vi "Boiler System Open.vi"(8 "error constant":errorcluster) -> (0 "error out":errorcluster, 1 "Configuration Data":T1, 2 "Notifiers":T5, 3 "Message Queues out":T6, 5 "User Event - Stop":refnum<user-event>, 7 "Stop Event Registration Refnum":refnum<event-registration>)   [LabVIEW 2017]
uses:
  Message Queue/All Message Queues.ctl
  Message Queue/Message Cluster.ctl
  Notifieres/Notifiers.ctl
  Configuration/Configuration Data.ctl
  controls/MHL Configuration.ctl
  Controller/Controller Configuration.ctl
  Boiler/Boiler Configuration.ctl
  User Event - Stop/User Event - Stop.lvlib
  Message Queue/Message Queue.lvlib
  Controller/Controller.lvlib
  Boiler/Boiler.lvlib
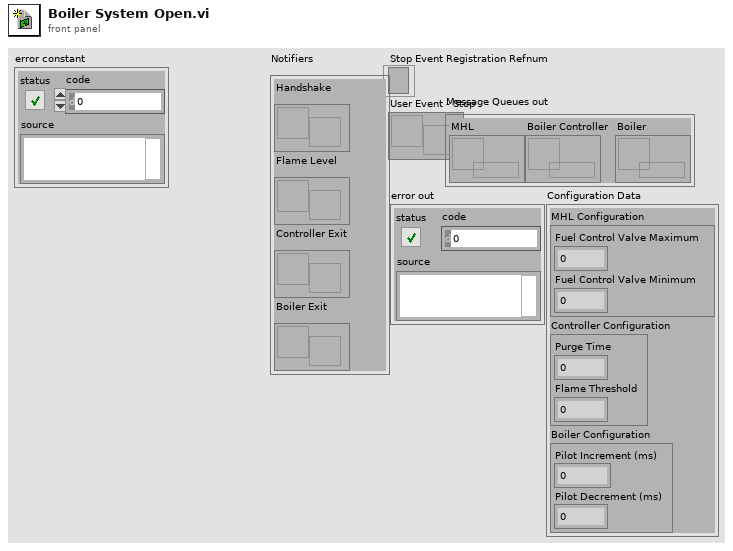
[diagram p1: front panel]
types:
  T1 = typedef "Configuration Data.ctl" = cluster{"MHL Configuration":T2, "Controller Configuration":T3, "Boiler Configuration":T4}
  T2 = typedef "MHL Configuration.ctl" = cluster{"Fuel Control Valve Maximum":dbl, "Fuel Control Valve Minimum":dbl}
  T3 = typedef "Controller.lvlib/Controller Configuration.ctl" = cluster{"Purge Time":u32, "Flame Threshold":u32}
  T4 = typedef "Boiler.lvlib/Boiler Configuration.ctl" = cluster{"Pilot Increment (ms)":u32, "Pilot Decrement (ms)":u32}
  T5 = typedef "Notifiers.ctl" = cluster{"Handshake":refnum<notifier>, "Flame Level":refnum<notifier>, "Controller Exit":refnum<notifier>, "Boiler Exit":refnum<notifier>}
  T6 = typedef "Message Queue.lvlib/All Message Queues.ctl" = cluster{"MHL":refnum<queue>, "Boiler Controller":refnum<queue>, "Boiler":refnum<queue>}
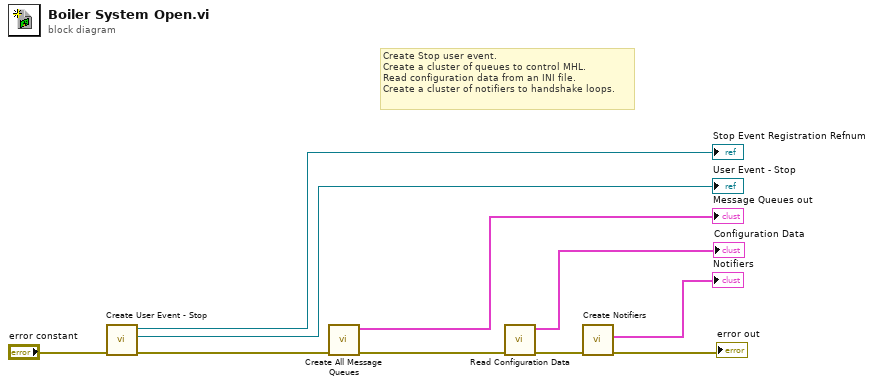
[diagram p0: block diagram]
diagram:
  # "Create Stop user event.\nCreate a cluster of queues to control MHL.\nRead configuration data from an INI file.\nCreate a cluster of notifiers to handshake loops."
  n1 = call "Create User Event - Stop.vi"("error in (no error)"="error constant") -> ("error out"=w7:errorcluster, "User Event - Stop"=→"User Event - Stop":refnum<user-event>, "Stop Event Registration Refnum"=→"Stop Event Registration Refnum":refnum<event-registration>)  [unwired: 8 in]
  n2 = call "Create All Message Queues.vi"("error in (no error)"=w7) -> ("error out"=w3:errorcluster, "Message Queues out"=→"Message Queues out":T6)  [unwired: 9 in]
  n3 = call "Read Configuration Data.vi"("error in (no error)"=w3) -> ("error out"=w2:errorcluster, "Configuration Data"=→"Configuration Data":T1)  [unwired: 9 in]
  n4 = call "Create Notifiers.vi"("error constant"=w2) -> ("error out"=→"error out":errorcluster, "output cluster"=→"Notifiers":T5)  [unwired: 9 in]
